vi "TestRUSHShoot.vi"() -> ()   [LabVIEW 2012]
panel:
  out "Out Cluster":T1
  in  "Set 3":bool
  in  "Set 2":bool
  in  "Set 1":bool
  in  "In Cluster":T2
  in  "ShootConstElev":cluster{"1":dbl, "2":dbl, "3":dbl}={"1"=45.0, "2"=24.0, "3"=12.0}
  in  "ShootTargetInfo":T3
  in  "Deadband":dbl=0.1
  in  "Default Wheel Speed":dbl=0.75
  in  "IndexerSpeed":dbl=0.5
  in  "ShootManualElev":dbl(slide) scale=-1.0..1.0
  in  "ShootPOTElev":dbl(slide) scale=0.0..45.0
  in  "ShootCase":dbl
  in  "ShootIndexerEnable":bool
  in  "ShootStartWheels":bool
  in  "ShootTrackEnable":bool
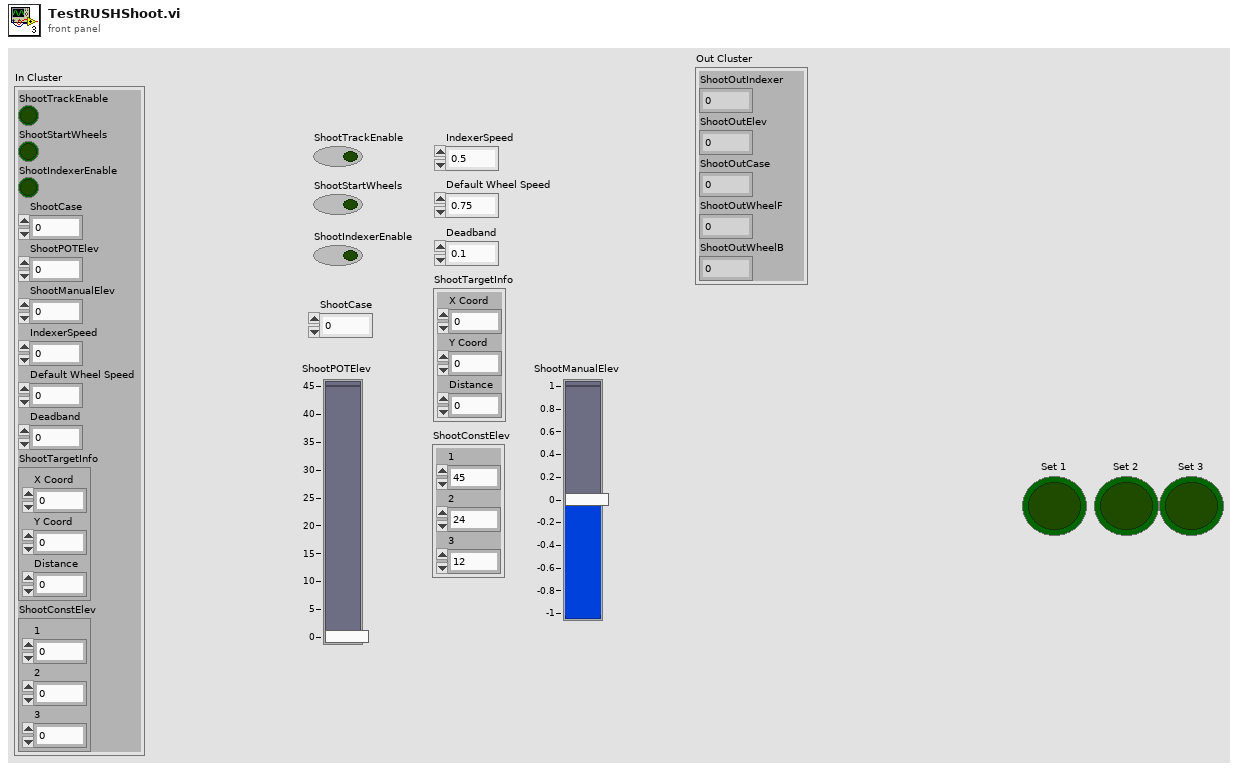
[diagram p1: front panel]
types:
  T1 = cluster{"ShootOutIndexer":dbl, "ShootOutElev":dbl, "ShootOutCase":dbl, "ShootOutWheelF":dbl, "ShootOutWheelB":dbl}
  T2 = cluster{"ShootTrackEnable":bool, "ShootStartWheels":bool, "ShootIndexerEnable":bool, "ShootCase":dbl, "ShootPOTElev":dbl, "ShootManualElev":dbl, "IndexerSpeed":dbl, "Default Wheel Speed":dbl, "Deadband":dbl, "ShootTargetInfo":cluster{"X Coord":dbl, "Y Coord":dbl, "Distance":dbl}, "ShootConstElev":cluster{"1":dbl, "2":dbl, "3":dbl}}
  T3 = cluster{"X Coord":dbl, "Y Coord":dbl, "Distance":dbl}
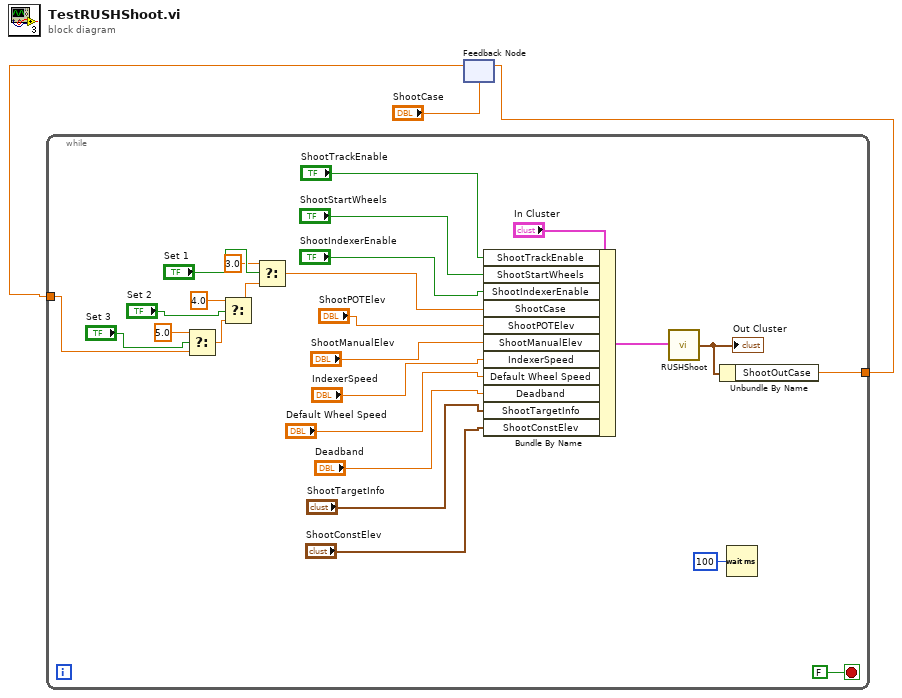
[diagram p0: block diagram]
diagram:
  n1 = feedback #1("ShootCase") -> (w3:dbl)
  n2 = while {
    tunnel: w3 -> [w21]
    tunnel: [w5] -> w1
    stop <- FALSE stop-if-true
    n3 = Select(t=5.0, s="Set 3", f=w21) -> (s? t:f=w23:dbl)
    n4 = Select(t=4.0, s="Set 2", f=w23) -> (s? t:f=w22:dbl)
    n5 = Select(t=3.0, s="Set 1", f=w22) -> (s? t:f=w17:dbl)
    n6 = Bundle By Name(cluster="In Cluster", "ShootTrackEnable"="ShootTrackEnable", "ShootStartWheels"="ShootStartWheels", "ShootIndexerEnable"="ShootIndexerEnable", "ShootCase"=w17, "ShootPOTElev"="ShootPOTElev", "ShootManualElev"="ShootManualElev", "IndexerSpeed"="IndexerSpeed", "Default Wheel Speed"="Default Wheel Speed", "Deadband"="Deadband", "ShootTargetInfo"="ShootTargetInfo", "ShootConstElev"="ShootConstElev") -> (w26:T2)
    n7 = call "RUSHShoot.vi"("In Cluster"=w26) -> ("Out Cluster"=w6:T1)
    "Out Cluster" <- w6
    n8 = Unbundle By Name(w6) -> ("ShootOutCase"=w5:dbl)
    n9 = Wait (ms)(milliseconds to wait=u32 100) -> ()  [unwired: 1 out]
  }
  n10 = feedback-in #1(w1) -> ()
